vi "Sample.vi"() -> ()   [LabVIEW 2010]
panel:
  out "Width":i32
  out "Height":i32
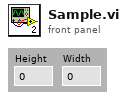
[diagram p1: front panel]
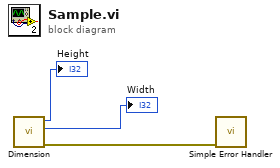
[diagram p0: block diagram]
diagram:
  n1 = call "Dimension.vi"() -> ("error out"=w1:errorcluster, "Width"=→"Width":i32, "Height"=→"Height":i32)  [unwired: 9 in]
  n2 = call <vilib>:"Simple Error Handler.vi"("error in (no error)"=w1) -> ()  [unwired: 4 in, 5 out]
